vi "Load_ConfigCoude.vi"(8 "error in":errorcluster) -> (0 "error out":errorcluster, 2 "Resp":string)   [LabVIEW 2011]
uses:
  Global Coude.vi
  <vilib>/Utility/config.llb/NI_LVConfig.lvlib
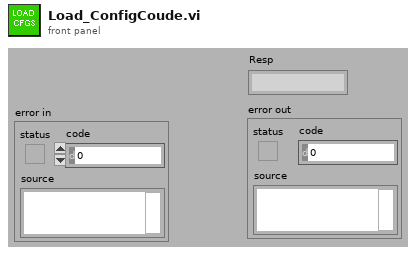
[diagram p1: front panel]
types:
  T1 = cluster{"Mec ID":string, "VISA Mec":refnum<visa-resource-name>, "Mec PosLimit":string, "Mec NegLimit":string, "Mec Factor":dbl, "Mec Speed":dbl, "Mec Acceleration":dbl, "MecOffset":string, "MecTargets":dbl[], "MecEnabled":bool, "Mec Target":dbl}
  T2 = typedef "NI_LVConfig.lvlib/Config Data RefNum.ctl" = refnum<k1>
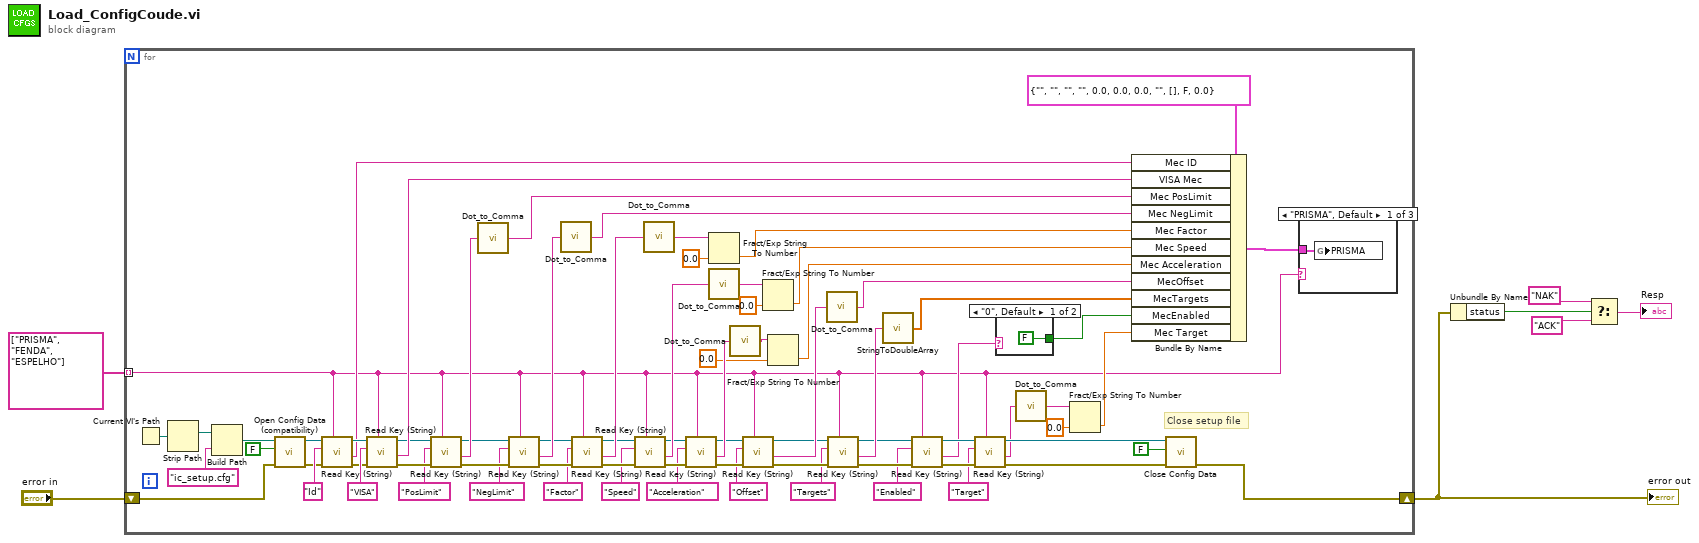
[diagram p0: block diagram]
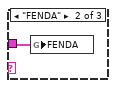
[diagram p2: hidden frame]
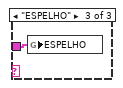
[diagram p3: hidden frame]
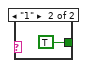
[diagram p4: hidden frame]
diagram:
  n1 = for {
    tunnel: string[] ["PRISMA", "FENDA", "ESPELHO"] -> [w10] mode=indexing
    shift-right: [w8] -> w5
    shift-left: "error in" -> [w9]
    # "Close setup file"
    n2 = Current VI's Path() -> (path=w35:path)
    n3 = Strip Path(path=w35) -> (stripped path=w36:path)  [unwired: 1 out]
    n4 = Build Path(base path=w36, name or relative path="ic_setup.cfg") -> (appended path=w16:path)
    n5 = call <vilib>:"Open Config Data (compatibility).vi"("error in (no error)"=w9, "create file if necessary (T)"=FALSE ("create file if necessary? (T)"), "configuration file path"=w16) -> ("error out"=w14:errorcluster, "refnum"=w13:T2)  [unwired: 6 in, 1 out]
    n6 = call <vilib>:"Read Key (String).vi"("section"=w10, "error in (no error)"=w14, "key"="Id", "refnum"=w13) -> ("error out"=w18:errorcluster, "value"=w17:string, "refnum out"=w19:T2)  [unwired: 2 in, 3 out]
    n7 = call <vilib>:"Read Key (String).vi"("section"=w10, "error in (no error)"=w18, "key"="VISA", "refnum"=w19) -> ("error out"=w60:errorcluster, "value"=w74:string, "refnum out"=w56:T2)  [unwired: 2 in, 3 out]
    n8 = call <vilib>:"Read Key (String).vi"("section"=w10, "error in (no error)"=w60, "key"="PosLimit", "refnum"=w56) -> ("error out"=w62:errorcluster, "value"=w66:string, "refnum out"=w61:T2)  [unwired: 2 in, 3 out]
    n9 = call "Dot_to_Comma.vi"("String in"=w66) -> ("String out"=w75:string)
    n10 = call <vilib>:"Read Key (String).vi"("section"=w10, "error in (no error)"=w62, "key"="NegLimit", "refnum"=w61) -> ("error out"=w59:errorcluster, "value"=w67:string, "refnum out"=w55:T2)  [unwired: 2 in, 3 out]
    n11 = call "Dot_to_Comma.vi"("String in"=w67) -> ("String out"=w76:string)
    n12 = call <vilib>:"Read Key (String).vi"("section"=w10, "error in (no error)"=w59, "key"="Factor", "refnum"=w55) -> ("error out"=w58:errorcluster, "value"=w68:string, "refnum out"=w54:T2)  [unwired: 2 in, 3 out]
    n13 = call <vilib>:"Read Key (String).vi"("section"=w10, "error in (no error)"=w58, "key"="Speed", "refnum"=w54) -> ("error out"=w57:errorcluster, "value"=w64:string, "refnum out"=w53:T2)  [unwired: 2 in, 3 out]
    n14 = call "Dot_to_Comma.vi"("String in"=w68) -> ("String out"=w69:string)
    n15 = call <vilib>:"Read Key (String).vi"("section"=w10, "error in (no error)"=w57, "key"="Acceleration", "refnum"=w53) -> ("error out"=w48:errorcluster, "value"=w70:string, "refnum out"=w47:T2)  [unwired: 2 in, 3 out]
    n16 = Fract/Exp String To Number(string=w69, default (0 dbl)=0.0 ("default (0 DBL)")) -> (number=w77:dbl)  [unwired: 3 out]
    n17 = call "Dot_to_Comma.vi"("String in"=w64) -> ("String out"=w65:string)
    n18 = call "Dot_to_Comma.vi"("String in"=w70) -> ("String out"=w71:string)
    n19 = call <vilib>:"Read Key (String).vi"("section"=w10, "error in (no error)"=w48, "key"="Offset", "refnum"=w47) -> ("error out"=w46:errorcluster, "value"=w72:string, "refnum out"=w45:T2)  [unwired: 2 in, 3 out]
    n20 = Fract/Exp String To Number(string=w65, default (0 dbl)=0.0) -> (number=w78:dbl)  [unwired: 3 out]
    n21 = Fract/Exp String To Number(string=w71, default (0 dbl)=0.0) -> (number=w79:dbl)  [unwired: 3 out]
    n22 = call "Dot_to_Comma.vi"("String in"=w72) -> ("String out"=w80:string)
    n23 = call <vilib>:"Read Key (String).vi"("section"=w10, "error in (no error)"=w46, "key"="Targets", "refnum"=w45) -> ("error out"=w31:errorcluster, "value"=w38:string, "refnum out"=w34:T2)  [unwired: 2 in, 3 out]
    n24 = call "StringToDoubleArray.vi"("String"=w38) -> ("MecTargets"=w81:dbl[])
    n25 = call <vilib>:"Read Key (String).vi"("section"=w10, "error in (no error)"=w31, "key"="Enabled", "refnum"=w34) -> ("error out"=w30:errorcluster, "value"=w26:string, "refnum out"=w33:T2)  [unwired: 2 in, 3 out]
    n26 = call <vilib>:"Read Key (String).vi"("section"=w10, "error in (no error)"=w30, "key"="Target", "refnum"=w33) -> ("error out"=w29:errorcluster, "value"=w22:string, "refnum out"=w32:T2)  [unwired: 2 in, 3 out]
    n27 = case shown="\"0\", Default" w26 {
      tunnel: [FALSE TRUE] -> w25
      frame "0", Default {
      }
      frame "1" {
      }
    }
    n28 = call "Dot_to_Comma.vi"("String in"=w22) -> ("String out"=w24:string)
    n29 = Fract/Exp String To Number(string=w24, default (0 dbl)=0.0) -> (number=w21:dbl)  [unwired: 3 out]
    n30 = Bundle By Name(cluster=T1 {"Mec ID"="", "VISA Mec"="", "Mec PosLimit"="", "Mec NegLimit"="", "Mec Factor"=0.0, "Mec Speed"=0.0, "Mec Acceleration"=0.0, "MecOffset"="", "MecTargets"=[], "MecEnabled"=FALSE, "Mec Target"=0.0} ("CAM"), "Mec ID"=w17, "VISA Mec"=w74, "Mec PosLimit"=w75, "Mec NegLimit"=w76, "Mec Factor"=w77, "Mec Speed"=w78, "Mec Acceleration"=w79, "MecOffset"=w80, "MecTargets"=w81, "MecEnabled"=w25, "Mec Target"=w21) -> (w12:T1)
    n31 = call <vilib>:"Close Config Data.vi"("error in (no error)"=w29, "write file if changed (T)"=FALSE ("create file if necessary? (T)"), "refnum"=w32) -> ("error out"=w8:errorcluster)  [unwired: 8 out]
    n32 = case shown="\"PRISMA\", Default" w10 {
      tunnel: w12 -> [w82 w83 w84]
      frame "PRISMA", Default {
        n33 = global write "Global Coude.vi" "PRISMA"(w82) -> ()
      }
      frame "FENDA" {
        n34 = global write "Global Coude.vi" "FENDA"(w83) -> ()
      }
      frame "ESPELHO" {
        n35 = global write "Global Coude.vi" "ESPELHO"(w84) -> ()
      }
    }
  }
  "error out" <- w5
  n36 = Unbundle By Name(w5) -> ("status"=w4:bool)
  n37 = Select(t="NAK", s=w4, f="ACK") -> (s? t:f=→"Resp":string)
